vi "DN4_AI_ReadData.vi"(4 "error IO":errorcluster, 5 "count":i32, 7 "Task ID":u32) -> (0 "error out":errorcluster, 1 "data":dbl[](array[numeric]), 2 "start time":dbl, 3 "Task ID":u32)   [LabVIEW 2009]
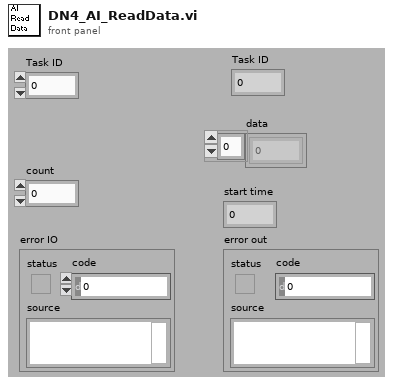
[diagram p1: front panel]
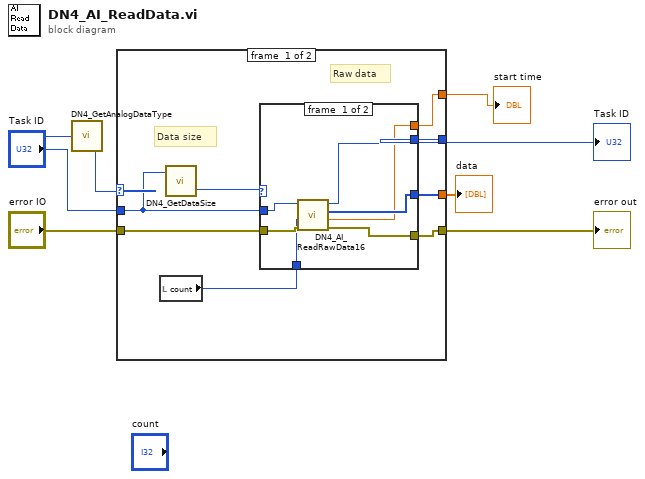
[diagram p0: block diagram]
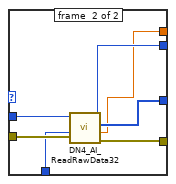
[diagram p2: hidden frame]
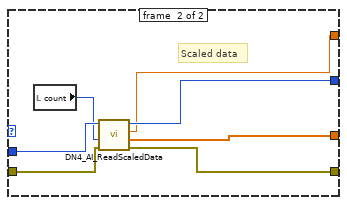
[diagram p3: hidden frame]
diagram:
  n1 = call <userlib>:"DN4_GetAnalogDataType.vi"("Task ID"="Task ID") -> ("return type"=w2:i32)
  n2 = case shown="1, Default" w2 {
    tunnel: "Task ID" -> [w11 w36]
    tunnel: "error IO" -> [w15 w35]
    tunnel: [w9 w34] -> w5
    tunnel: [w13 w32] -> w7
    tunnel: [w14 w33] -> w6
    tunnel: [w8 w30] -> w1
    frame #0 {
      # "Raw data"
      # "Data size"
      n3 = local read "count"() -> (w12:i32)
      n4 = call <userlib>:"DN4_GetDataSize.vi"("Task ID"=w11) -> ("return type"=w10:i32)  [unwired: 2 out]
      n5 = case shown="4" w10 {
        tunnel: w15 -> [w21 w29]
        tunnel: [w20 w28] -> w14
        tunnel: w11 -> [w22 w27]
        tunnel: [w19 w26] -> w13
        tunnel: w12 -> [w18 w25]
        tunnel: [w17 w24] -> w9
        tunnel: [w16 w23] -> w8
        frame #0 {
          n6 = call <userlib>:"DN4_AI_ReadRawData16.vi"("Task ID"=w22, "count"=w18, "error in (no error)"=w21) -> ("Task ID"=w20:u32, "data"=w19:u16[], "start time"=w16:dbl, "error out"=w17:errorcluster)  [unwired: 1 in, 3 out]
        }
        frame #1 {
          n7 = call <userlib>:"DN4_AI_ReadRawData32.vi"("Task ID"=w27, "count"=w25, "error in (no error)"=w29) -> ("Task ID"=w28:u32, "data"=w26:u32[], "start time"=w23:dbl, "error out"=w24:errorcluster)  [unwired: 1 in, 3 out]
        }
      }
    }
    frame #1 {
      # "Scaled data"
      n8 = local read "count"() -> (w31:i32)
      n9 = call <userlib>:"DN4_AI_ReadScaledData.vi"("error in (no error)"=w35, "count"=w31, "Task ID"=w36) -> ("error out"=w34:errorcluster, "data"=w32:dbl[], "start time"=w30:dbl, "Task ID"=w33:u32)  [unwired: 1 out]
    }
  }
  "data" <- w7
  "Task ID" <- w6
  "error out" <- w5
  "start time" <- w1
